vi "DMM_Scan PRD 32V-16C Configure and Measure.vi"(0 "Scan Resources Handles In":T2={"DMM Handle"="", "MUX Handle"="", "Relays Debounce Time (ms)"=5, "Close all Shunts?"=TRUE}, 5 "Scan Configuration":T3[](array[typedef]) {"Resolution in Digits" items=["3 1/2"=3.5, "4 1/2"=4.5, "5 1/2"=5.5, "6 1/2"=6.5, "7 1/2"=7.5]}, 11 "error in":errorcluster) -> (4 "Scan Resources Handles Out":T1={"DMM Handle"="", "MUX Handle"="", "Relays Debounce Time (ms)"=5, "Close all Shunts?"=TRUE}, 6 "Formatted Measurements":T6[](array[typedef]) {"Switch Time" format="%#_3p"}, 8 "Raw Measurements":T5[](array[typedef]) {"Value" format="%#_8g"}, 10 "Execution Settings":T7[](array[typedef]) {"Function" items=["DC Volts"=1, "AC Volts"=2, "DC Current"=3, "AC Current"=4, "2-Wire Resistance"=5, "4-Wire Resistance"=101, "Frequency"=104, "Period"=105, "AC Volts DC Coupled"=1001, "Diode"=1002, "Waveform Voltage"=1003, "Waveform Current"=1004, "Capacitance"=1005, "Inductance"=1006, "Temperature"=108]; "Absolute\nResolution" format="%#_6p"; "Input Resistance\n(Ohm)" format="%#_6p"; "Range" format="%#_6p"; "Minimum\nFrequency (Hz)" format="%#_6p"; "Aperture\nTime (s)" format="%#_6p"; "Auto Range\nValue" format="%#_6p"; "Settle\nTime (s)" format="%#_6p"}, 14 "Total Scan Time (s)":dbl format="%#.3p", 15 "error out":errorcluster)   [LabVIEW 2021, in "DMM_Scan PXI RLY Driver 32V-16C.lvlib"]
doc: "Configures an NI-DMM Scan measurement list on the resource provided by the Scan Resource Handle In control according to each given channel number (ex. ch0, ch1), Function/Range, Digits. \n\nReturns Formatted Measurements based on Channels, Measurements (string with units), Out of Range, Individual Measurement Time (including configuration, aperture and relay debounce).\n\nReturns Raw Measurements (numeric values) to be used and compared in a sequencer.\n\nReturns Execution Settings and Total Scan Time (s) for optimization, debugging and reporting."
uses:
  DMM_Scan PXI RLY Driver 32V-16C.lvlib
  Typedefs/Scan configuration.ctl
  <instrlib>/niDMM/nidmm.llb/niDMM Resolution in Digits.ctl
  Typedefs/Measurement values.ctl
  Typedefs/Formatted measurement.ctl
  DMM Mixed Measurements/DMM Mixed Meas Typedefs/DMM Execution Settings.ctl
  Typedefs/Scan Resource Handles In.ctl
  Typedefs/Scan Resource Handles Out.ctl
  DMM Mixed Measurements/DMM Mixed Meas Typedefs/Function Settings.ctl
  Static Digital Path Generation/Typedefs/Terminal and State Settings.ctl
  Common/Typedefs/Execution Options - Measure.ctl
  DMM Mixed Measurements/DMM_Mixed Measurement.lvlib
  Static Digital Path Generation/Switch_Static Digital Path Generation.lvlib
panel:
  # "Inputs"
  # "Outputs"
  # "Channels"
  # "Functions/Range"
  # "Digits"
  # "Channels"
  # "Values"
  # "Units"
  # "Out of R."
  # "Channels"
  # "Measurements"
  # "Out of."
  # "Time"
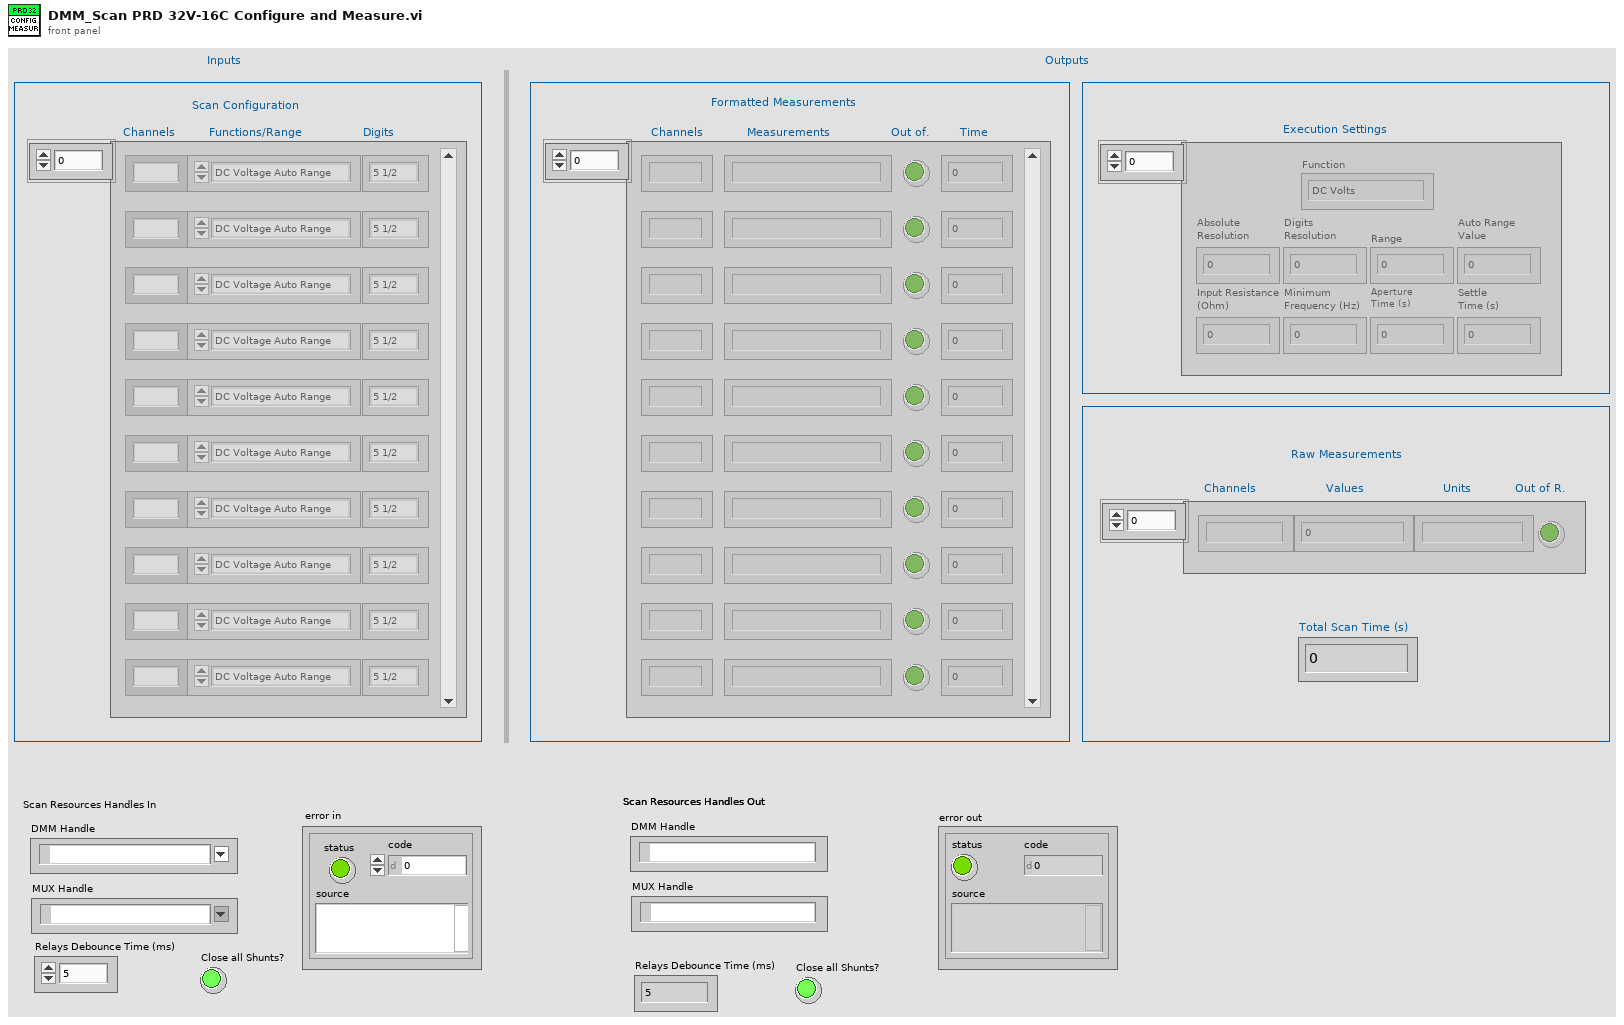
[diagram p1: front panel]
types:
  T1 = typedef "DMM_Scan PXI RLY Driver 32V-16C.lvlib/Scan Resource Handles Out.ctl" = cluster{"DMM Handle":refnum<k15>, "MUX Handle":refnum<k15>, "Relays Debounce Time (ms)":u32, "Close all Shunts?":bool}
  T2 = typedef "DMM_Scan PXI RLY Driver 32V-16C.lvlib/Scan Resource Handles In.ctl" = cluster{"DMM Handle":refnum<k15>, "MUX Handle":refnum<k15>, "Relays Debounce Time (ms)":u32, "Close all Shunts?":bool}
  T3 = typedef "DMM_Scan PXI RLY Driver 32V-16C.lvlib/Scan configuration.ctl" = cluster{"Channel":string, "Resolution in Digits":T4, "Range and Function":enum16{"DC Voltage Auto Range", "DC 100 mV", "DC 1 V ", "DC 10 V", "DC 100 V", "DC 300 V", " ", "AC Voltage Auto Range", "AC 50 mV", "AC 200 mV", "AC 500 mV", "AC 2 V", "AC 5 V", "AC 20 V", "AC 50 V", "AC 300 V", "  ", "DC Current Auto Range", "DC 1 uA", "DC 10 uA", "DC 100 uA", "DC 1 mA", "DC 10 mA", "DC 20 mA", "DC 100 mA", "DC 200 mA", "DC 1 A", "DC 3 A", "   ", "AC Current Auto Range", "AC 100 uA", "AC 1 mA", "AC 10 mA", "AC 100 mA", "AC 500 mA", "AC 1 A", "AC 3 A", "    ", "Resistance Auto Range", "Res 100 Ohm", "Res 1 kOhm", "Res 10 kOhm", "Res 100 kOhm", "Res 1 MOhm", "Res 10 MOhm", "Res 100 MOhm", "Res 5 GOhm", "     ", "Frequency AC Auto Range", "Freq AC 50 mV", "Freq AC 500 mV", "Freq AC 5 V", "Freq AC 50 V", "Freq AC 300 V", "      ", "Period AC Auto Range", "Period AC 50 mV", "Period AC 500 mV", "Period AC 5 V", "Period AC 50 V", "Period AC 300 V"}}
  T4 = typedef "niDMM Resolution in Digits.ctl" = dbl
  T5 = typedef "DMM_Scan PXI RLY Driver 32V-16C.lvlib/Measurement values.ctl" = cluster{"Channel":string, "Value":dbl, "Unit":string, "Out of Range":bool}
  T6 = typedef "DMM_Scan PXI RLY Driver 32V-16C.lvlib/Formatted measurement.ctl" = cluster{"Channel":string, "Switch Time":dbl, "Formatted Measurement":string, "Out of Range":bool}
  T7 = typedef "DMM_Mixed Measurement.lvlib/DMM Execution Settings.ctl" = cluster{"Absolute\nResolution":dbl, "Input Resistance\n(Ohm)":dbl, "Digits\nResolution":dbl, "Range":dbl, "Minimum\nFrequency (Hz)":dbl, "Aperture\nTime (s)":dbl, "Auto Range\nValue":dbl, "Settle\nTime (s)":dbl, "Function":i32}
  T8 = typedef "DMM_Mixed Measurement.lvlib/Function Settings.ctl" = cluster{"Range and Function":enum16{"DC Voltage Auto Range", "DC 100 mV", "DC 1 V ", "DC 10 V", "DC 100 V", "DC 300 V", " ", "AC Voltage Auto Range", "AC 50 mV", "AC 200 mV", "AC 500 mV", "AC 2 V", "AC 5 V", "AC 20 V", "AC 50 V", "AC 300 V", "  ", "DC Current Auto Range", "DC 1 uA", "DC 10 uA", "DC 100 uA", "DC 1 mA", "DC 10 mA", "DC 20 mA", "DC 100 mA", "DC 200 mA", "DC 1 A", "DC 3 A", "   ", "AC Current Auto Range", "AC 100 uA", "AC 1 mA", "AC 10 mA", "AC 100 mA", "AC 500 mA", "AC 1 A", "AC 3 A", "    ", "Resistance Auto Range", "Res 100 Ohm", "Res 1 kOhm", "Res 10 kOhm", "Res 100 kOhm", "Res 1 MOhm", "Res 10 MOhm", "Res 100 MOhm", "Res 5 GOhm", "     ", "Frequency AC Auto Range", "Freq AC 50 mV", "Freq AC 500 mV", "Freq AC 5 V", "Freq AC 50 V", "Freq AC 300 V", "      ", "Period AC Auto Range", "Period AC 50 mV", "Period AC 500 mV", "Period AC 5 V", "Period AC 50 V", "Period AC 300 V"}, "Resolution in Digits":T4}
  T9 = enum16{"DC Voltage Auto Range", "DC 100 mV", "DC 1 V ", "DC 10 V", "DC 100 V", "DC 300 V", " ", "AC Voltage Auto Range", "AC 50 mV", "AC 200 mV", "AC 500 mV", "AC 2 V", "AC 5 V", "AC 20 V", "AC 50 V", "AC 300 V", "  ", "DC Current Auto Range", "DC 1 uA", "DC 10 uA", "DC 100 uA", "DC 1 mA", "DC 10 mA", "DC 20 mA", "DC 100 mA", "DC 200 mA", "DC 1 A", "DC 3 A", "   ", "AC Current Auto Range", "AC 100 uA", "AC 1 mA", "AC 10 mA", "AC 100 mA", "AC 500 mA", "AC 1 A", "AC 3 A", "    ", "Resistance Auto Range", "Res 100 Ohm", "Res 1 kOhm", "Res 10 kOhm", "Res 100 kOhm", "Res 1 MOhm", "Res 10 MOhm", "Res 100 MOhm", "Res 5 GOhm", "     ", "Frequency AC Auto Range", "Freq AC 50 mV", "Freq AC 500 mV", "Freq AC 5 V", "Freq AC 50 V", "Freq AC 300 V", "      ", "Period AC Auto Range", "Period AC 50 mV", "Period AC 500 mV", "Period AC 5 V", "Period AC 50 V", "Period AC 300 V"}
  T10 = typedef "Execution Options - Measure.ctl" = enum16{"Configure & Measure", "Configure only", "Measure only"}
  T11 = typedef "Switch_Static Digital Path Generation.lvlib/Terminal and State Settings.ctl" = cluster{"Connect/Disconnect":bool, "Channel 1":string, "Channel 2":string}
  T12 = cluster{"Range and Function":bool, "Resolution in Digits":bool}
  T13 = typedef "DMM_Mixed Measurement.lvlib/Measurement.ctl" = cluster{"Measured Value":dbl, "Out of Range":bool, "Unit":string, "Measurement":string}
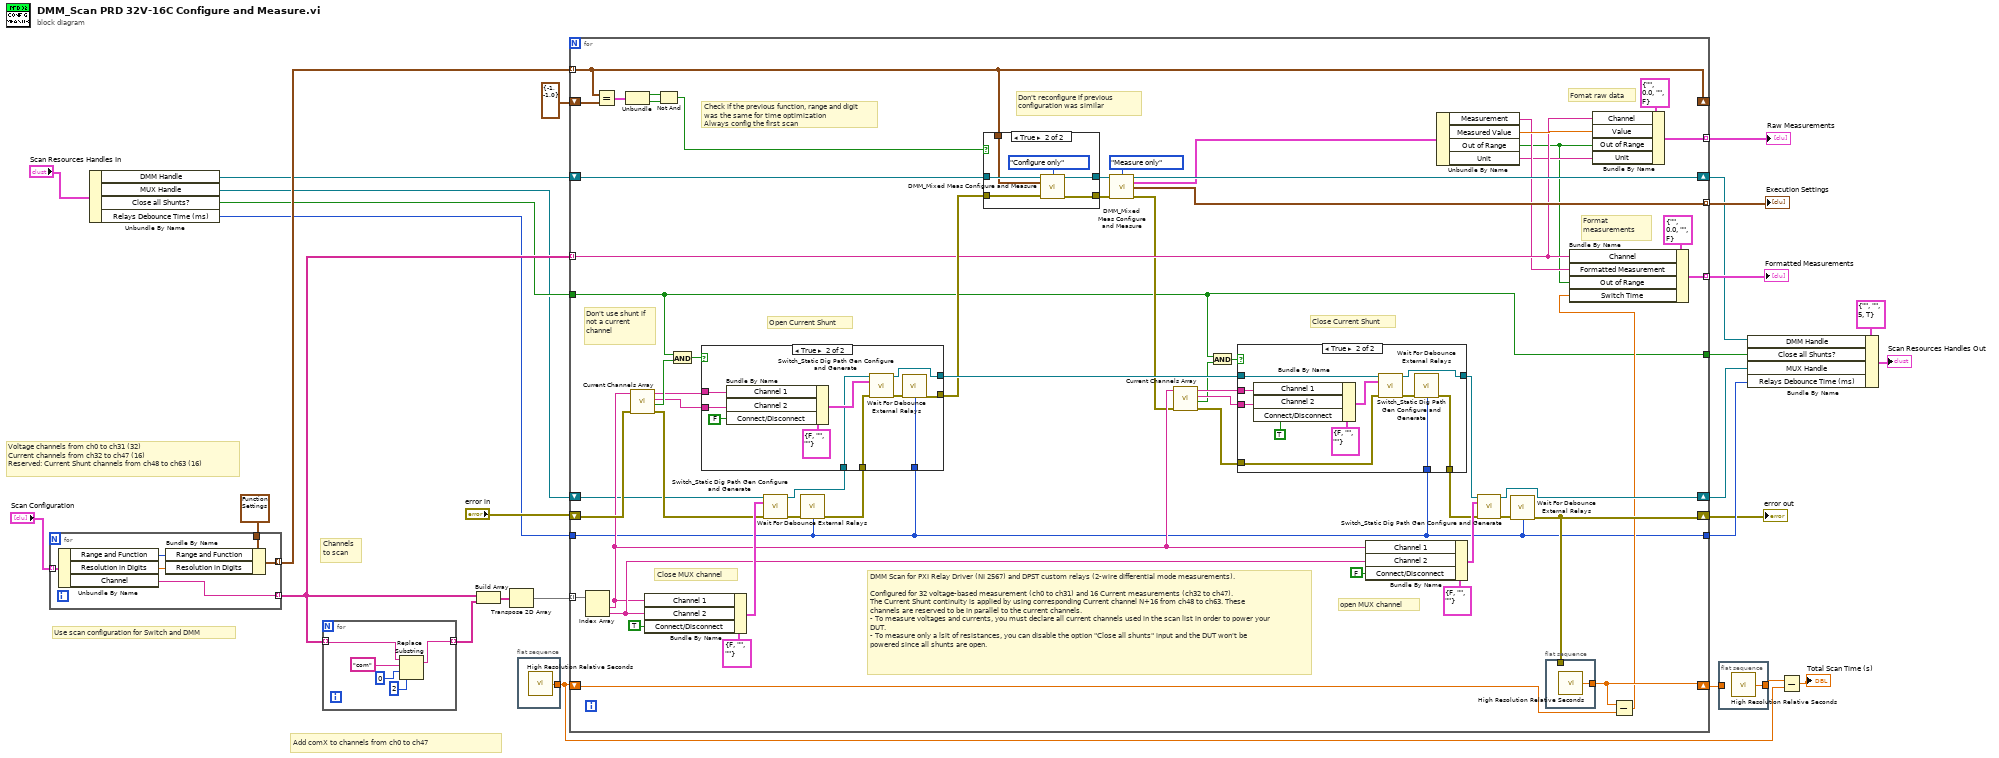
[diagram p0: block diagram]
diagram:
  # "Voltage channels from ch0 to ch31 (32)\nCurrent channels from ch32 to ch47 (16)\nReserved: Current Shunt channels from ch48 to ch63 (16)"
  # "Add comX to channels from ch0 to ch47"
  # "Use scan configuration for Switch and DMM"
  # "Channels\nto scan"
  n1 = for {
    tunnel: "Scan Configuration" -> [w33] mode=indexing
    tunnel: [w34] -> w20 mode=indexing
    tunnel: [w31] -> w28 mode=indexing
    tunnel: T8 {"Range and Function"=enum."DC Voltage Auto Range", "Resolution in Digits"=5.5} ("Function Settings") -> [w29]
    n2 = Unbundle By Name(w33) -> ("Range and Function"=w30:T9, "Resolution in Digits"=w32:T4, "Channel"=w34:string)
    n3 = Bundle By Name(cluster=w29, "Range and Function"=w30, "Resolution in Digits"=w32) -> (w31:T8)
  }
  n4 = Unbundle By Name("Scan Resources Handles In") -> ("DMM Handle"=w15:refnum<k15>, "MUX Handle"=w9:refnum<k15>, "Close all Shunts?"=w11:bool, "Relays Debounce Time (ms)"=w5:u32)
  n5 = for {
    tunnel: w20 -> [w36] mode=indexing
    tunnel: [w35] -> w12 mode=indexing
    n6 = Replace Substring(2:2 ("length (len. of substring)"), 3:0 ("offset (0)"), 4:"com" ("substring (\"\")"), 5:w36) -> (1:w35:string)  [unwired: 1 out]
  }
  n7 = Build Array(w20, w12) -> (w16:string[][])
  n8 = Transpose 2D Array(2D array=w16) -> (transposed array=w22:string[][])
  n9 = flat-sequence {
    tunnel: [w40] -> w25
    frame #0 {
      n10 = call <vilib>:"High Resolution Relative Seconds.vi"() -> ("relative seconds"=w40:dbl)
    }
  }
  n11 = for {
    shift-right: [w97] -> w14
    shift-left: w15 -> [w88]
    shift-right: [w45] -> w3
    shift-left: w9 -> [w50]
    shift-right: [w44] -> w1
    shift-left: "error in" -> [w62]
    tunnel: w22 -> [w96] mode=indexing
    shift-right: [w99] -> w26
    shift-left: w25 -> [w98]
    tunnel: w28 -> [w75] mode=indexing
    shift-right: [w75] -> _
    shift-left: cluster{i32, dbl} {-1, -1.0} -> [w79]
    tunnel: [w82] -> w17 mode=indexing
    tunnel: w20 -> [w69] mode=indexing
    tunnel: [w71] -> w19 mode=indexing
    tunnel: [w67] -> w18 mode=indexing
    tunnel: w11 -> [w42]
    tunnel: w5 -> [w41]
    tunnel: [w42] -> w4
    tunnel: [w41] -> w2
    # "DMM Scan for PXI Relay Driver (NI 2567) and DPST custom relays (2-wire differential mode measurements).\n\nConfigured for 32 voltage-based measurement (ch0 to ch31) and 16 Current measurements (ch32 to ch47).\nThe Current Shunt continuity is applied by using corresponding Current channel N+16 from ch48 to ch63. These channels are reserved to be in parallel to the current channels.\n- To measure voltages and currents, you must declare all current channels used in the scan list in order to power your DUT.\n- To measure only a lsit of resistances, you can disable the option \"Close all shunts\" input and the DUT won't be powered since all shunts are open."
    # "Don't use shunt if not a current channel"
    # "Format measurements"
    # "Fomat raw data"
    # "open MUX channel"
    # "Close MUX channel"
    # "Close Current Shunt"
    # "Open Current Shunt"
    # "Check if the previous function, range and digit was the same for time optimization\nAlways config the first scan"
    # "Don't reconfigure if previous configuration was similar"
    n12 = Index Array(array=w96) -> (element #1=w60:string, element #2=w92:string)  [unwired: 2 in]
    n13 = Equal?(x=w75, y=w79) -> (x = y?=w84:T12)
    n14 = Unbundle(w84) -> ("Range and Function"=w81:bool, "Resolution in Digits"=w80:bool)
    n15 = call "Current Channels Array.vi"("error in"=w62, "Channel 1"=w60) -> ("error out"=w61:errorcluster, "Current Channel?"=w57:bool, "Channel 2"=w55:string, "Channel 1"=w56:string)  [unwired: 6 in]
    n16 = Bundle By Name(cluster=T11 {"Connect/Disconnect"=FALSE, "Channel 1"="", "Channel 2"=""} ("Terminal and State Settings"), "Channel 1"=w60, "Channel 2"=w92, "Connect/Disconnect"=TRUE ("Connect Path")) -> (w95:T11)
    n17 = Not And(1:w80, 2:w81) -> (0:w83:bool)
    n18 = And(x=w42, y=w57) -> (x .and. y?=w64:bool)
    n19 = call "Switch_Static Dig Path Gen Configure and Generate.vi"("Switch Handle In"=w50, "Terminal and State Settings"=w95, "error in"=w61) -> ("Switch Handle Out"=w47:refnum<k15>, "error out"=w49:errorcluster)  [unwired: 10 in, 1 out]
    n20 = call "Wait For Debounce External Relays.vi"("error in"=w49, "Wait (ms)"=w41) -> ("error out"=w48:errorcluster)  [unwired: 13 in]
    n21 = case shown="True" w64 {
      tunnel: [w113 w116] -> w78
      tunnel: w48 -> [w114 w125]
      tunnel: [w114 w117] -> w77
      tunnel: w56 -> [_ w121]
      tunnel: w55 -> [_ w120]
      tunnel: w47 -> [w113 w119]
      tunnel: w41 -> [_ w115]
      frame False {
      }
      frame True {
        n22 = Bundle By Name(cluster=T11 {"Connect/Disconnect"=FALSE, "Channel 1"="", "Channel 2"=""} ("Terminal and State Settings"), "Channel 1"=w121, "Channel 2"=w120, "Connect/Disconnect"=FALSE) -> (w124:T11)
        n23 = call "Switch_Static Dig Path Gen Configure and Generate.vi"("Switch Handle In"=w119, "Terminal and State Settings"=w124, "error in"=w125) -> ("Switch Handle Out"=w116:refnum<k15>, "error out"=w118:errorcluster)  [unwired: 10 in, 1 out]
        n24 = call "Wait For Debounce External Relays.vi"("error in"=w118, "Wait (ms)"=w115) -> ("error out"=w117:errorcluster)  [unwired: 13 in]
      }
    }
    n25 = case shown="True" w83 {
      tunnel: w88 -> [w127 w133]
      tunnel: [w127 w132] -> w87
      tunnel: [w126 w130] -> w85
      tunnel: w75 -> [_ w128]
      tunnel: w77 -> [w126 w129]
      frame False {
      }
      frame True {
        n26 = call "DMM_Mixed Meas Configure and Measure.vi"("DMM Handle In"=w133, "Execution Option"=Execution_Options_-_Measure."Configure only", "Function Settings"=w128, "error in"=w129) -> ("DMM Handle Out"=w132:refnum<k15>, "error out"=w130:errorcluster)  [unwired: 8 in, 2 out]
      }
    }
    n27 = call "DMM_Mixed Meas Configure and Measure.vi"("DMM Handle In"=w87, "Execution Option"=Execution_Options_-_Measure."Measure only", "error in"=w85) -> ("DMM Handle Out"=w97:refnum<k15>, "Measurement"=w74:T13, "DMM Execution Settings"=w82:T7, "error out"=w59:errorcluster)  [unwired: 9 in]
    n28 = call "Current Channels Array.vi"("error in"=w59, "Channel 1"=w60) -> ("error out"=w58:errorcluster, "Current Channel?"=w52:bool, "Channel 2"=w53:string, "Channel 1"=w54:string)  [unwired: 6 in]
    n29 = And(x=w42, y=w52) -> (x .and. y?=w63:bool)
    n30 = case shown="True" w63 {
      tunnel: w78 -> [w101 w112]
      tunnel: [w101 w105] -> w51
      tunnel: [w100 w103] -> w76
      tunnel: w54 -> [_ w108]
      tunnel: w58 -> [w100 w107]
      tunnel: w53 -> [_ w106]
      tunnel: w41 -> [_ w102]
      frame False {
      }
      frame True {
        n31 = Bundle By Name(cluster=T11 {"Connect/Disconnect"=FALSE, "Channel 1"="", "Channel 2"=""} ("Terminal and State Settings"), "Channel 1"=w108, "Channel 2"=w106, "Connect/Disconnect"=TRUE) -> (w109:T11)
        n32 = call "Switch_Static Dig Path Gen Configure and Generate.vi"("Switch Handle In"=w112, "Terminal and State Settings"=w109, "error in"=w107) -> ("Switch Handle Out"=w105:refnum<k15>, "error out"=w104:errorcluster)  [unwired: 10 in, 1 out]
        n33 = call "Wait For Debounce External Relays.vi"("error in"=w104, "Wait (ms)"=w102) -> ("error out"=w103:errorcluster)  [unwired: 13 in]
      }
    }
    n34 = Bundle By Name(cluster=T11 {"Connect/Disconnect"=FALSE, "Channel 1"="", "Channel 2"=""} ("Terminal and State Settings"), "Channel 1"=w60, "Channel 2"=w92, "Connect/Disconnect"=FALSE ("Disconnect Path")) -> (w93:T11)
    n35 = Unbundle By Name(w74) -> ("Measurement"=w68:string, "Measured Value"=w72:dbl, "Out of Range"=w65:bool, "Unit"=w66:string)
    n36 = call "Switch_Static Dig Path Gen Configure and Generate.vi"("Switch Handle In"=w51, "Terminal and State Settings"=w93, "error in"=w76) -> ("Switch Handle Out"=w45:refnum<k15>, "error out"=w46:errorcluster)  [unwired: 10 in, 1 out]
    n37 = call "Wait For Debounce External Relays.vi"("error in"=w46, "Wait (ms)"=w41) -> ("error out"=w44:errorcluster)  [unwired: 13 in]
    n38 = flat-sequence {
      tunnel: [w134] -> w99
      tunnel: w44 -> [_]
      frame #0 {
        n39 = call <vilib>:"High Resolution Relative Seconds.vi"() -> ("relative seconds"=w134:dbl)
      }
    }
    n40 = Bundle By Name(cluster=T5 {"Channel"="", "Value"=0.0, "Unit"="", "Out of Range"=FALSE} ("Measurements"), "Channel"=w69, "Value"=w72, "Out of Range"=w65, "Unit"=w66) -> (w71:T5)
    n41 = Subtract(x=w99, y=w98) -> (x-y=w43:dbl)
    n42 = Bundle By Name(cluster=T6 {"Channel"="", "Switch Time"=0.0, "Formatted Measurement"="", "Out of Range"=FALSE} ("Measurements"), "Channel"=w69, "Formatted Measurement"=w68, "Out of Range"=w65, "Switch Time"=w43) -> (w67:T6)
  }
  "Raw Measurements" <- w19
  "Formatted Measurements" <- w18
  "Execution Settings" <- w17
  "error out" <- w1
  n43 = flat-sequence {
    tunnel: [w135] -> w24
    tunnel: w26 -> [_]
    frame #0 {
      n44 = call <vilib>:"High Resolution Relative Seconds.vi"() -> ("relative seconds"=w135:dbl)
    }
  }
  n45 = Bundle By Name(cluster=T1 {"DMM Handle"="", "MUX Handle"="", "Relays Debounce Time (ms)"=5, "Close all Shunts?"=TRUE} ("Scan Resources Handles Out"), "DMM Handle"=w14, "Close all Shunts?"=w4, "MUX Handle"=w3, "Relays Debounce Time (ms)"=w2) -> (→"Scan Resources Handles Out":T1)
  n46 = Subtract(x=w24, y=w25) -> (x-y=→"Total Scan Time (s)":dbl)
